vi "D6 Datalog Main.vi"(8 "error in":errorcluster, 11 "Queue Ref":T1) -> ()   [LabVIEW 2022 SP3]
uses:
  Controls/All Queue Ref.ctl
  Controls/D6 Root path.ctl
  Controls/Log main.ctl
  Controls/ALL Health.ctl
  6D_Global.vi
  <vilib>/Waveform/WDTOps.llb/WDT Get Waveform Time Array DBL.vi
  <vilib>/Waveform/DWDTOps.llb/DWDT Get Waveform Time Array.vi
  <vilib>/Waveform/DWDTOps.llb/DWDT Digital to Analog.vi
panel:
  out "error in":errorcluster
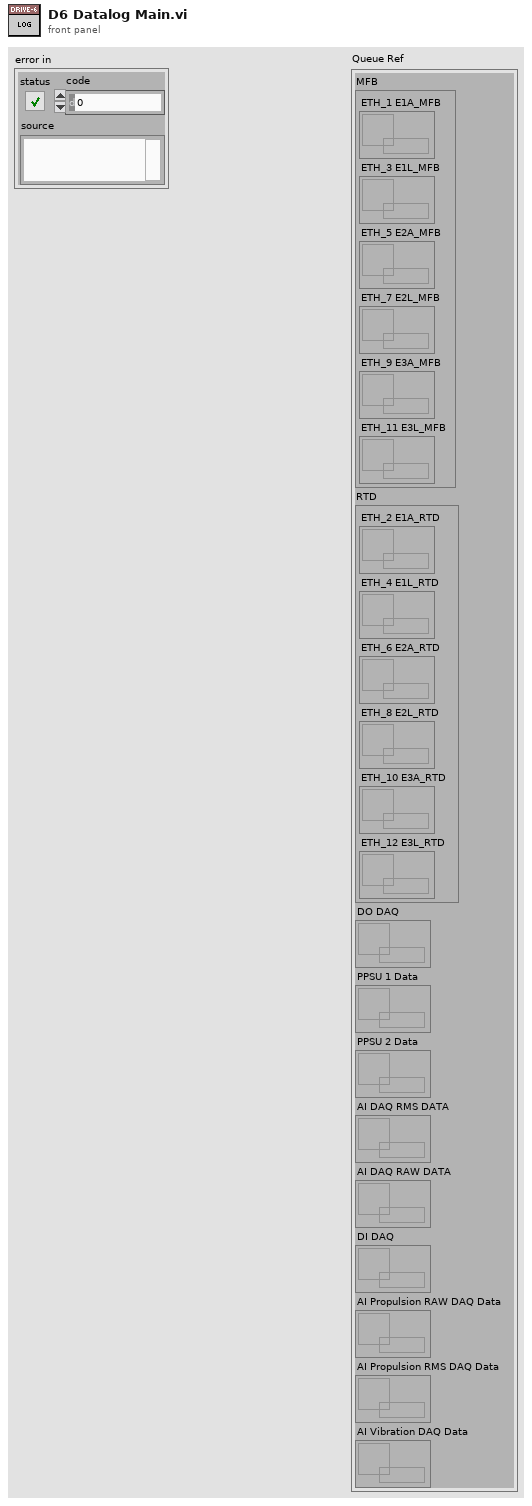
[diagram p1: front panel]
types:
  T1 = typedef "All Queue Ref.ctl" = cluster{"MFB":cluster{"ETH_1 E1A_MFB":refnum<queue>, "ETH_3 E1L_MFB":refnum<queue>, "ETH_5 E2A_MFB":refnum<queue>, "ETH_7 E2L_MFB":refnum<queue>, "ETH_9 E3A_MFB":refnum<queue>, "ETH_11 E3L_MFB":refnum<queue>}, "RTD":cluster{"ETH_2 E1A_RTD ":refnum<queue>, "ETH_4 E1L_RTD ":refnum<queue>, "ETH_6 E2A_RTD ":refnum<queue>, "ETH_8 E2L_RTD ":refnum<queue>, "ETH_10 E3A_RTD ":refnum<queue>, "ETH_12 E3L_RTD ":refnum<queue>}, "DO DAQ":refnum<queue>, "PPSU 1 Data":refnum<queue>, "PPSU 2 Data":refnum<queue>, "AI DAQ RMS DATA":refnum<queue>, "AI DAQ RAW DATA":refnum<queue>, "DI DAQ":refnum<queue>, "AI Propulsion RAW DAQ Data":refnum<queue>, "AI Propulsion RMS DAQ Data":refnum<queue>, "AI Vibration DAQ Data":refnum<queue>}
  T2 = typedef "Log main.ctl" = enum16{"Init", "Poll", "Flush Qs", "Create File", "PPSU Data", "Log MFB", "Log RTD", "Log DO", "Log AI RAW", "Log AI RMS", "Log AI RMS Propulsion", "Log AI RAW Propulsion ", "Log AI Vibration", "Log DI", "Close File", "Error", "Exit"}
  T3 = typedef "D6 Root path.ctl" = cluster{"Data":path, "Sub VI's":path, "Source code":path}
  T4 = cluster{"in progress?":bool, "tdms ref":refnum<k34>, "Start time":timestamp, "Root Path":T3, "Queue Ref":T1}
  T5 = enum16{"open", "open or create", "create or replace", "create", "open (read-only)"}
  T6 = typedef "ALL Health.ctl" = enum16{"AI HS", "AI Vibration HS", "AI Propulsion HS", "DO HS", "Datalog HS", "PPSU HS", "ETH_1 DAQ", "ETH_1 RTD", "ETH_2 DAQ", "ETH_2 RTD", "ETH_5 RTD"}
  T7 = enum16{"Init", "Read 'All'", "Read 'n'", "Read '1'", "Write '1'", "Write 'n'", "Write 'All'"}
  T8 = cluster{"ETH_1 E1A_MFB":refnum<queue>, "ETH_3 E1L_MFB":refnum<queue>, "ETH_5 E2A_MFB":refnum<queue>, "ETH_7 E2L_MFB":refnum<queue>, "ETH_9 E3A_MFB":refnum<queue>, "ETH_11 E3L_MFB":refnum<queue>}
  T9 = cluster{"ETH_2 E1A_RTD ":refnum<queue>, "ETH_4 E1L_RTD ":refnum<queue>, "ETH_6 E2A_RTD ":refnum<queue>, "ETH_8 E2L_RTD ":refnum<queue>, "ETH_10 E3A_RTD ":refnum<queue>, "ETH_12 E3L_RTD ":refnum<queue>}
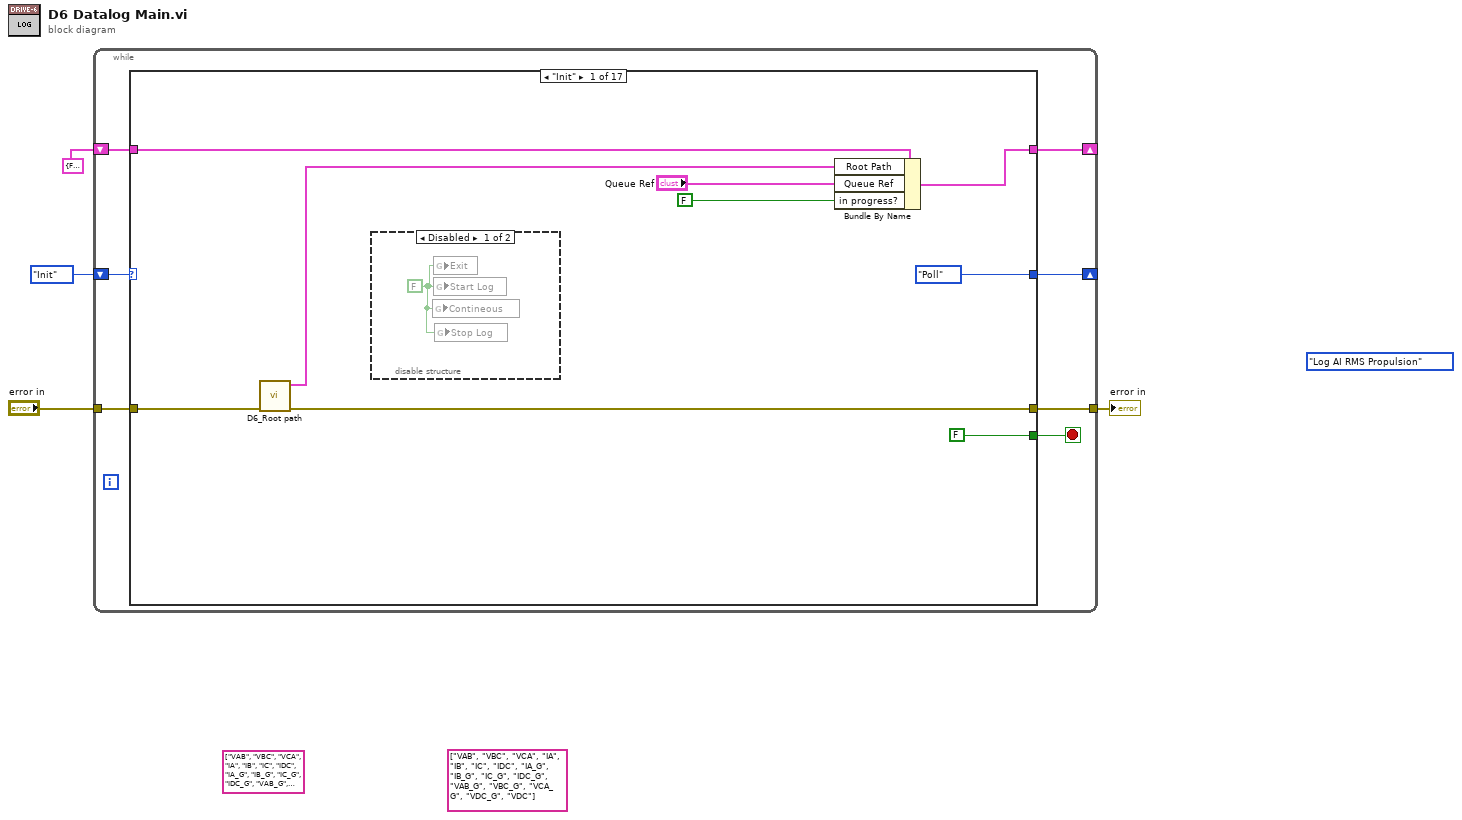
[diagram p0: block diagram]
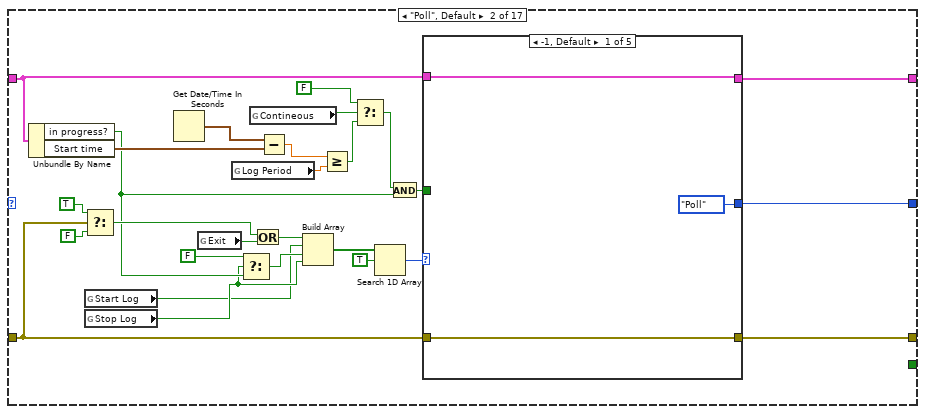
[diagram p3: hidden frame]
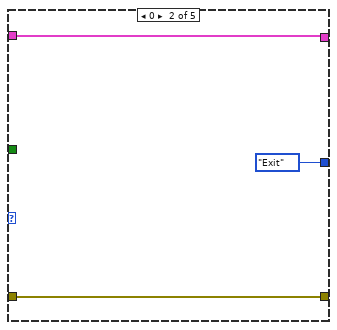
[diagram p4: hidden frame]
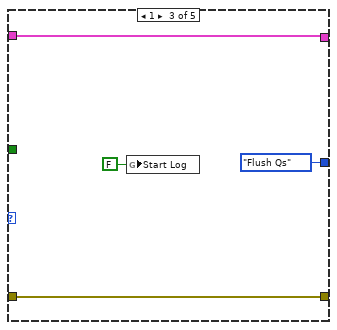
[diagram p5: hidden frame]
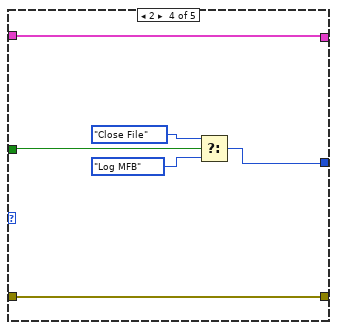
[diagram p6: hidden frame]
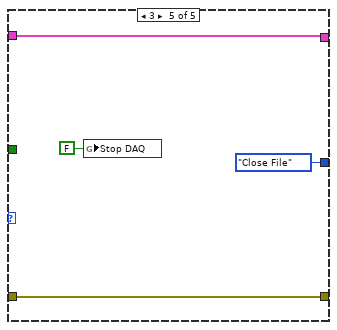
[diagram p7: hidden frame]
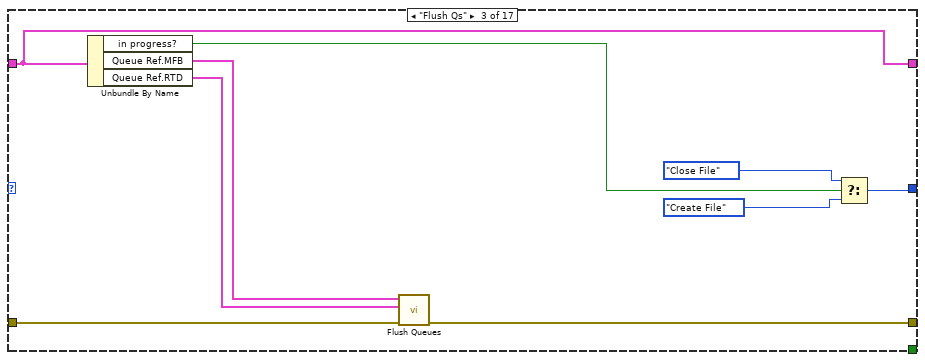
[diagram p8: hidden frame]
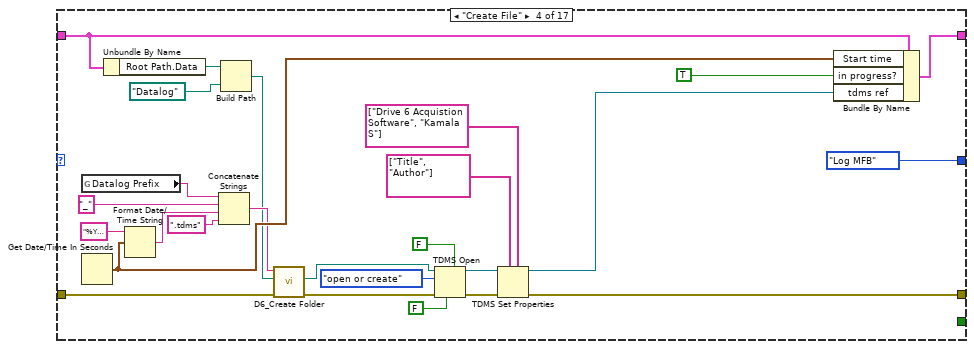
[diagram p9: hidden frame]
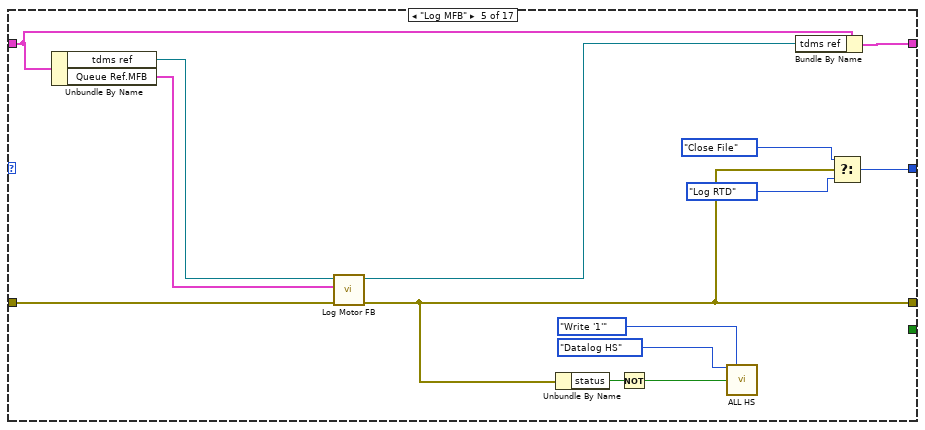
[diagram p10: hidden frame]
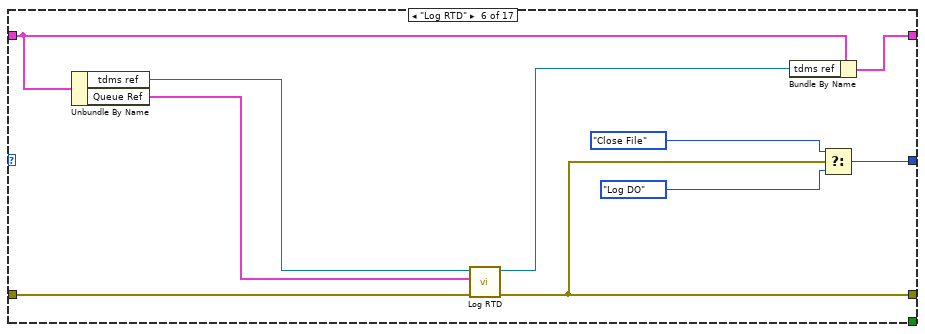
[diagram p11: hidden frame]
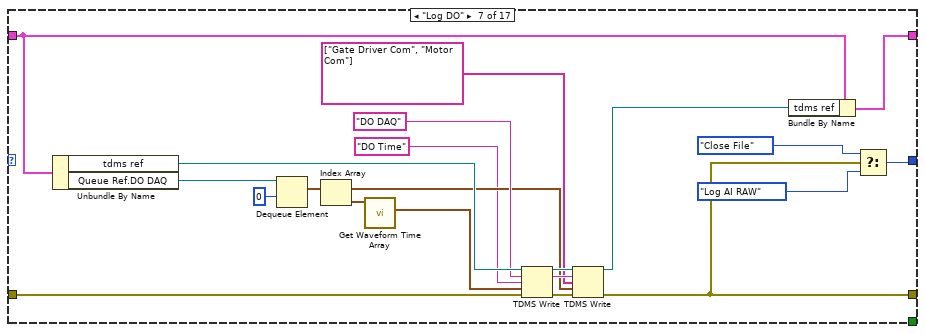
[diagram p12: hidden frame]
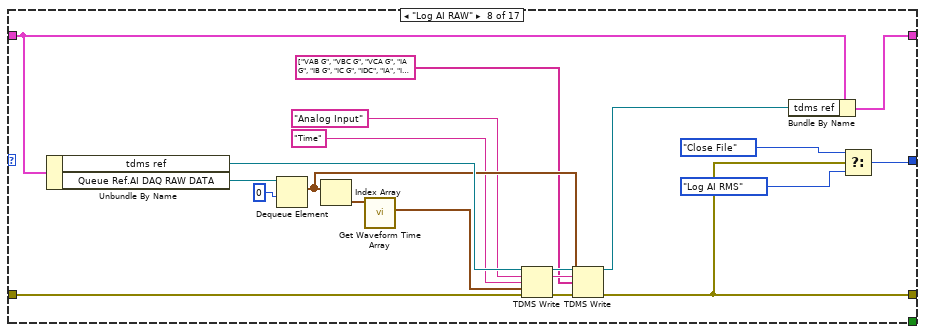
[diagram p13: hidden frame]
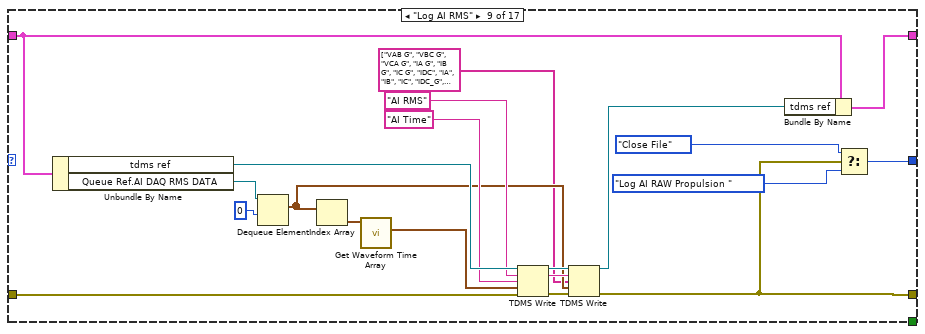
[diagram p14: hidden frame]
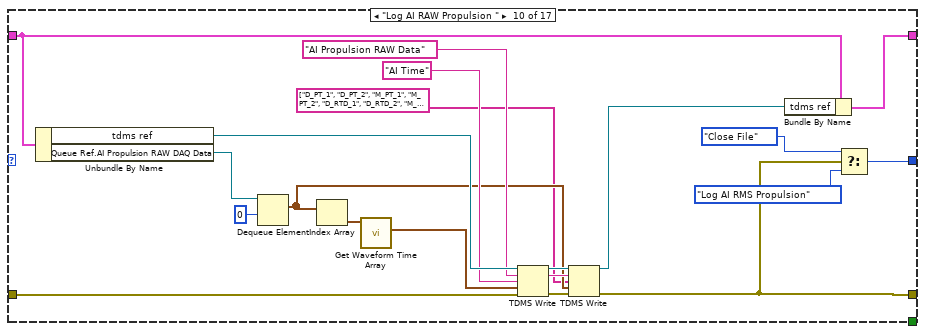
[diagram p15: hidden frame]
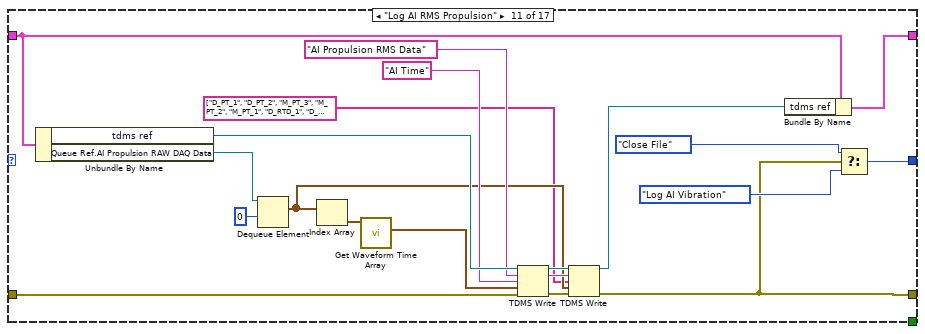
[diagram p16: hidden frame]
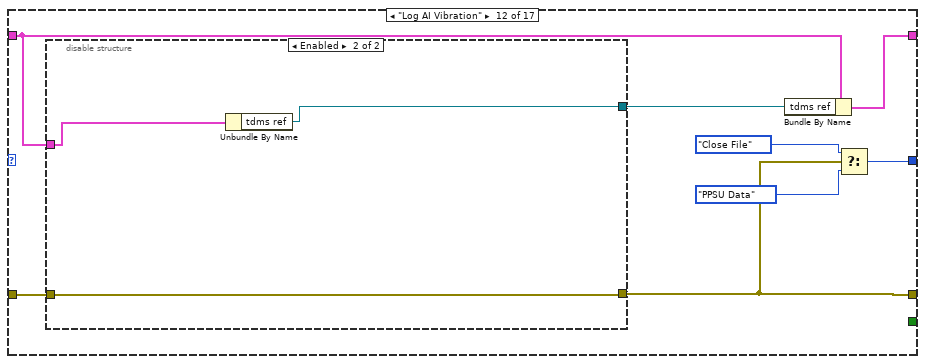
[diagram p17: hidden frame]
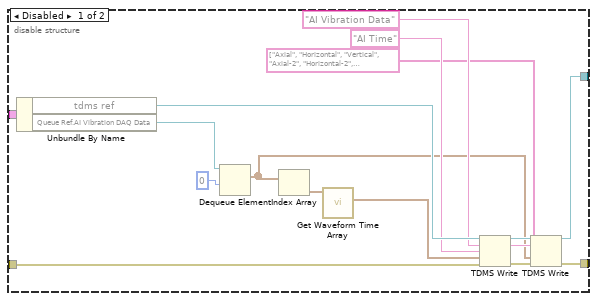
[diagram p18: hidden frame]
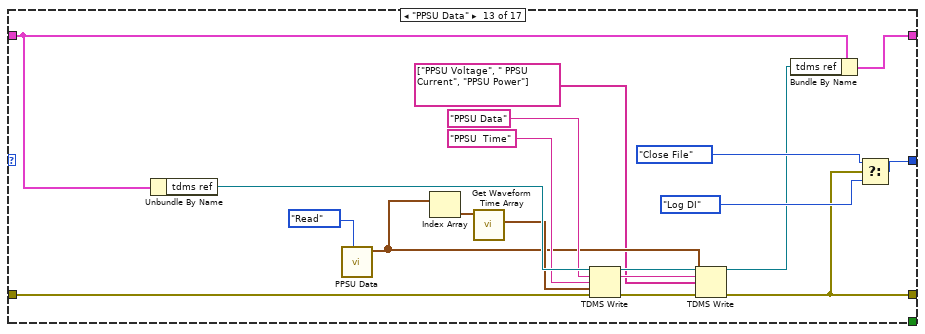
[diagram p19: hidden frame]
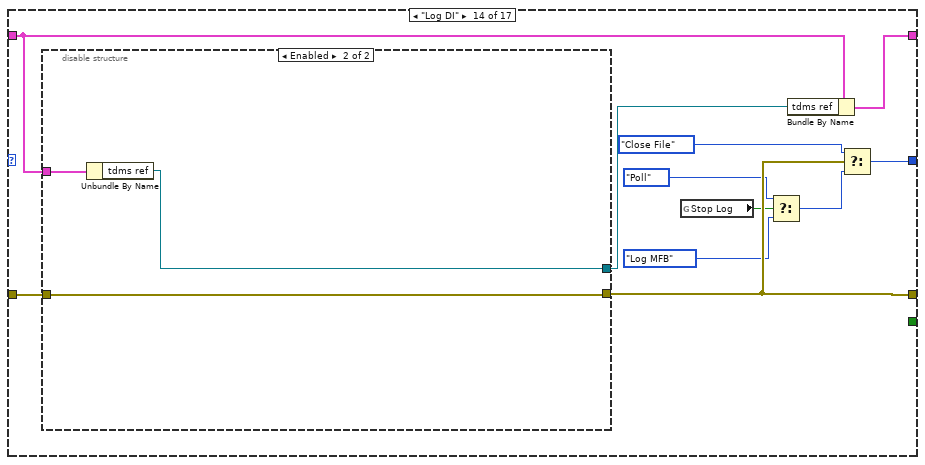
[diagram p20: hidden frame]
diagram:
  (unwired) string[] ["VAB", "VBC", "VCA", "IA", "IB", "IC", "IDC", "IA_G", "IB_G", "IC_G", "IDC_G", "VAB_G", "VBC_G", "VCA_G", "VDC_G", "VDC"] ("channel name(s) in (Untitled)")
  (unwired) string[] ["VAB", "VBC", "VCA", "IA", "IB", "IC", "IDC", "IA_G", "IB_G", "IC_G", "IDC_G", "VAB_G", "VBC_G", "VCA_G", "VDC_G", "VDC"] ("channel name(s) in (Untitled)")
  (unwired) Log_main."Log AI RMS Propulsion"
  n1 = while {
    shift-right: [w10] -> _
    shift-left: Log_main."Init" -> [w11]
    shift-right: [w7] -> _
    shift-left: T4 {"in progress?"=FALSE, "tdms ref"=refnum, "Start time"=timestamp(0 s since 1904-01-01), "Root Path"={"Data"=path "", "Sub VI's"=path "", "Source code"=path ""}, "Queue Ref"={"MFB"={"ETH_1 E1A_MFB"=refnum, "ETH_3 E1L_MFB"=refnum, "ETH_5 E2A_MFB"=refnum, "ETH_7 E2L_MFB"=refnum, "ETH_9 E3A_MFB"=refnum, "ETH_11 E3L_MFB"=refnum}, "RTD"={"ETH_2 E1A_RTD "=refnum, "ETH_4 E1L_RTD "=refnum, "ETH_6 E2A_RTD "=refnum, "ETH_8 E2L_RTD "=refnum, "ETH_10 E3A_RTD "=refnum, "ETH_12 E3L_RTD "=refnum}, "DO DAQ"=refnum, "PPSU 1 Data"=refnum, "PPSU 2 Data"=refnum, "AI DAQ RMS DATA"=refnum, "AI DAQ RAW DATA"=refnum, "DI DAQ"=refnum, "AI Propulsion RAW DAQ Data"=refnum, "AI Propulsion RMS DAQ Data"=refnum, "AI Vibration DAQ Data"=refnum}} -> [w8]
    tunnel: "error in" -> [w6]
    tunnel: [w5] -> w2
    stop <- w9 stop-if-true
    n2 = case shown="\"Init\"" w11 {
      tunnel: [Log_main."Poll" w48 w77 Log_main."Log MFB" w115 w125 w143 w161 w175 w201 w220 w228 w260 w280 Log_main."Exit" w322 Log_main."Close File"] -> w10
      tunnel: [FALSE _ _ _ _ _ _ _ _ _ _ _ _ _ TRUE _ TRUE] -> w9
      tunnel: w8 -> [w19 w45 w75 w90 w116 w126 w146 w164 w177 w203 w222 w230 w259 w279 w311 w324 w335]
      tunnel: [w20 w46 w75 w93 w117 w127 w145 w163 w176 w202 w221 w229 w258 w278 w311 w325 w335] -> w7
      tunnel: w6 -> [w18 w24 w74 w84 w112 w122 w147 w165 w178 w204 w223 w231 w255 w282 w310 w327 w336]
      tunnel: [w16 w47 w71 w78 w106 w121 w141 w159 w179 w205 w224 w232 w261 w281 w310 w326 w336] -> w5
      frame "Init" {
        n3 = call "D6_Root path.vi"("error in (no error)"=w18) -> ("error out"=w16:errorcluster, "Root Path"=w17:T3)  [unwired: 9 in]
        n4 = disable-structure shown="Disabled" {
          frame Disabled {
            w21 = FALSE ("Exit")
            n5 = global write "6D_Global.vi" "Contineous"(w21) -> ()
            n6 = global write "6D_Global.vi" "Exit"(w21) -> ()
            n7 = global write "6D_Global.vi" "Start Log"(w21) -> ()
            n8 = global write "6D_Global.vi" "Stop Log"(w21) -> ()
          }
          frame Enabled {
          }
        }
        n9 = Bundle By Name(cluster=w19, "Root Path"=w17, "Queue Ref"="Queue Ref", "in progress?"=FALSE) -> (w20:T4)
      }
      frame "Poll", Default {
        n10 = Unbundle By Name(w45) -> ("in progress?"=w26:bool, "Start time"=w36:timestamp)
        n11 = Select(t=TRUE, s=w24, f=FALSE) -> (s? t:f=w35:bool)
        n12 = global read "6D_Global.vi" "Start Log"() -> (w22:bool)
        n13 = global read "6D_Global.vi" "Stop Log"() -> (w23:bool)
        n14 = Get Date/Time In Seconds() -> (seconds since 1Jan1904=w37:timestamp)
        n15 = global read "6D_Global.vi" "Exit"() -> (w33:bool)
        n16 = global read "6D_Global.vi" "Log Period"() -> (w32:dbl)
        n17 = Select(t=FALSE ("Stop Log"), s=w23, f=w26) -> (s? t:f=w25:bool)
        n18 = global read "6D_Global.vi" "Contineous"() -> (w31:bool)
        n19 = Or(x=w35, y=w33) -> (x .or. y?=w34:bool)
        n20 = Subtract(x=w37, y=w36) -> (x-y=w39:dbl)
        n21 = Build Array(w34, w22, w25, w23) -> (w42:bool[])
        n22 = Greater Or Equal?(x=w39, y=w32) -> (x >= y?=w30:bool)
        n23 = Select(t=FALSE, s=w31, f=w30) -> (s? t:f=w29:bool)
        n24 = Search 1D Array(1D array=w42, element=TRUE) -> (index of element=w43:i32)  [unwired: 1 in]
        n25 = And(x=w29, y=w26) -> (x .and. y?=w38:bool)
        n26 = case shown="-1, Default" w43 {
          tunnel: [Log_main."Poll" Log_main."Exit" Log_main."Flush Qs" w59 Log_main."Close File"] -> w48
          tunnel: w24 -> [w50 w53 w58 w63 w66]
          tunnel: [w50 w53 w58 w63 w66] -> w47
          tunnel: [w51 w54 w57 w64 w67] -> w46
          tunnel: w45 -> [w51 w54 w57 w64 w67]
          tunnel: w38 -> [_ _ _ w62 _]
          frame -1, Default {
          }
          frame 0 {
          }
          frame 1 {
            n27 = global write "6D_Global.vi" "Start Log"(FALSE ("Start Log")) -> ()
          }
          frame 2 {
            n28 = Select(t=Log_main."Close File", s=w62, f=Log_main."Log MFB") -> (s? t:f=w59:T2)
          }
          frame 3 {
            n29 = global write "6D_Global.vi" "Stop DAQ"(FALSE ("Stop DAQ")) -> ()
          }
        }
      }
      frame "Flush Qs" {
        n30 = Unbundle By Name(w75) -> ("in progress?"=w76:bool, "Queue Ref.MFB"=w73:T8, "Queue Ref.RTD"=w72:T9)
        n31 = call "Flush Queues.vi"("error in"=w74, "RTD"=w72, "MFB"=w73) -> ("error out"=w71:errorcluster)  [unwired: 8 in]
        n32 = Select(t=Log_main."Close File", s=w76, f=Log_main."Create File") -> (s? t:f=w77:T2)
      }
      frame "Create File" {
        n33 = global read "6D_Global.vi" "Datalog Prefix"() -> (w85:string)
        n34 = Get Date/Time In Seconds() -> (seconds since 1Jan1904=w87:timestamp)
        n35 = Unbundle By Name(w90) -> ("Root Path.Data"=w89:path)
        n36 = Format Date/Time String(time format string (%c)="%Y_%b_%d_%Hh_%Mm_%Ssec", seconds (now)=w87) -> (date/time string=w97:string)  [unwired: 1 in]
        n37 = Concatenate Strings(w85, "_" ("string"), w97, ".tdms" ("string")) -> (w82:string)
        n38 = Build Path(base path=w89, name or relative path=path "Datalog" ("base path")) -> (appended path=w81:path)
        n39 = call "D6_Create Folder.vi"("error in (no error)"=w84, "Base Path"=w81, "File Name"=w82) -> ("error out"=w83:errorcluster, "Result File path"=w80:path)  [unwired: 6 in, 1 out]
        n40 = TDMS Open(5:FALSE ("create index file? (T)"), 6:FALSE ("disable buffering? (T)"), 8:w83, 10:T5."open or create" ("operation (0:open)"), 11:w80) -> (0:w102:errorcluster, 3:w103:refnum<k34>)  [unwired: 2 in]
        n41 = TDMS Set Properties(5:string[] ["Drive 6 Acquistion Software", "Kamala S"] ("property names"), 7:string[] ["Title", "Author"] ("property names"), 8:w102, 11:w103) -> (0:w78:errorcluster, 3:w91:refnum<k34>)  [unwired: 4 out]
        n42 = Bundle By Name(cluster=w90, "Start time"=w87, "in progress?"=TRUE, "tdms ref"=w91) -> (w93:T4)
      }
      frame "Log MFB" {
        n43 = Unbundle By Name(w116) -> ("tdms ref"=w111:refnum<k34>, "Queue Ref.MFB"=w109:T8)
        n44 = call "Log Motor FB.vi"("error in"=w112, "MFB"=w109, "tdms file in"=w111) -> ("error out"=w106:errorcluster, "tdms file in"=w110:refnum<k34>)  [unwired: 7 in]
        n45 = Unbundle By Name(w106) -> ("status"=w105:bool)
        n46 = Not(x=w105) -> (.not. x?=w104:bool)
        n47 = call "ALL HS.vi"("Loop"=ALL_Health."Datalog HS", "Option"=T7."Write '1'", "Status"=w104) -> ()  [unwired: 10 in, 3 out]
        n48 = Bundle By Name(cluster=w116, "tdms ref"=w110) -> (w117:T4)
        n49 = Select(t=Log_main."Close File", s=w106, f=Log_main."Log RTD") -> (s? t:f=w115:T2)
      }
      frame "Log RTD" {
        n50 = Unbundle By Name(w126) -> ("tdms ref"=w120:refnum<k34>, "Queue Ref"=w118:T1)
        n51 = call "Log RTD.vi"("error in 2"=w122, "Queue Ref"=w118, "tdms file in 2"=w120) -> ("error out 2"=w121:errorcluster, "tdms file in"=w119:refnum<k34>)  [unwired: 7 in]
        n52 = Bundle By Name(cluster=w126, "tdms ref"=w119) -> (w127:T4)
        n53 = Select(t=Log_main."Close File", s=w121, f=Log_main."Log DO") -> (s? t:f=w125:T2)
      }
      frame "Log DO" {
        n54 = Unbundle By Name(w146) -> ("tdms ref"=w139:refnum<k34>, "Queue Ref.DO DAQ"=w138:refnum<queue>)
        n55 = Dequeue Element(queue=w138, timeout in ms (-1)=0) -> (element=w130:waveform(dbl)[])  [unwired: 1 in, 3 out]
        n56 = Index Array(array=w130) -> (element=w137:waveform(dbl))  [unwired: 1 in]
        n57 = call-poly <vilib>:"Get Waveform Time Array.vi"("waveform in"=w137) -> ("X array"=w135:timestamp[])  [unwired: 9 in, 1 out]
        n58 = TDMS Write(0:w139, 5:"DO DAQ" ("group name in (Untitled)"), 7:"DO Time" ("group name in (Untitled)"), 9:w135, 11:w147) -> (4:w133:refnum<k34>, 6:w136:string, 15:w134:errorcluster)  [unwired: 1 in, 1 out]
        n59 = TDMS Write(0:w133, 5:w136, 7:string[] ["Gate Driver Com", "Motor Com"] ("channel name(s) in (Untitled)"), 9:w130, 11:w134) -> (4:w144:refnum<k34>, 15:w141:errorcluster)  [unwired: 1 in, 2 out]
        n60 = Bundle By Name(cluster=w146, "tdms ref"=w144) -> (w145:T4)
        n61 = Select(t=Log_main."Close File", s=w141, f=Log_main."Log AI RAW") -> (s? t:f=w143:T2)
      }
      frame "Log AI RAW" {
        n62 = Unbundle By Name(w164) -> ("tdms ref"=w167:refnum<k34>, "Queue Ref.AI DAQ RAW DATA"=w166:refnum<queue>)
        n63 = Dequeue Element(queue=w166, timeout in ms (-1)=0) -> (element=w152:waveform(dbl)[])  [unwired: 1 in, 3 out]
        n64 = Index Array(array=w152) -> (element=w158:waveform(dbl))  [unwired: 1 in]
        n65 = call-poly <vilib>:"Get Waveform Time Array.vi"("waveform in"=w158) -> ("X array"=w156:timestamp[])  [unwired: 9 in, 1 out]
        n66 = TDMS Write(0:w167, 5:"Analog Input" ("group name in (Untitled)"), 7:"Time" ("group name in (Untitled)"), 9:w156, 11:w165) -> (4:w154:refnum<k34>, 6:w157:string, 15:w155:errorcluster)  [unwired: 1 in, 1 out]
        n67 = TDMS Write(0:w154, 5:w157, 7:string[] ["VAB G", "VBC G", "VCA G", "IA G", "IB G", "IC G", "IDC", "IA", "IB", "IC", "IDC_G", "VAB", "VBC", "VCA", "VDC_G", "VDC"] ("channel name(s) in (Untitled)"), 9:w152, 11:w155) -> (4:w162:refnum<k34>, 15:w159:errorcluster)  [unwired: 1 in, 2 out]
        n68 = Bundle By Name(cluster=w164, "tdms ref"=w162) -> (w163:T4)
        n69 = Select(t=Log_main."Close File", s=w159, f=Log_main."Log AI RMS") -> (s? t:f=w161:T2)
      }
      frame "Log AI RMS" {
        n70 = Unbundle By Name(w177) -> ("tdms ref"=w187:refnum<k34>, "Queue Ref.AI DAQ RMS DATA"=w171:refnum<queue>)
        n71 = Dequeue Element(queue=w171, timeout in ms (-1)=0) -> (element=w170:waveform(dbl)[])  [unwired: 1 in, 3 out]
        n72 = Index Array(array=w170) -> (element=w184:waveform(dbl))  [unwired: 1 in]
        n73 = call-poly <vilib>:"Get Waveform Time Array.vi"("waveform in"=w184) -> ("X array"=w182:timestamp[])  [unwired: 9 in, 1 out]
        n74 = TDMS Write(0:w187, 5:"AI RMS" ("group name in (Untitled)"), 7:"AI Time" ("group name in (Untitled)"), 9:w182, 11:w178) -> (4:w180:refnum<k34>, 6:w183:string, 15:w181:errorcluster)  [unwired: 1 in, 1 out]
        n75 = TDMS Write(0:w180, 5:w183, 7:string[] ["VAB G", "VBC G", "VCA G", "IA G", "IB G", "IC G", "IDC", "IA", "IB", "IC", "IDC_G", "VAB", "VBC", "VCA", "VDC_G", "VDC"] ("channel name(s) in (Untitled)"), 9:w170, 11:w181) -> (4:w186:refnum<k34>, 15:w179:errorcluster)  [unwired: 1 in, 2 out]
        n76 = Bundle By Name(cluster=w177, "tdms ref"=w186) -> (w176:T4)
        n77 = Select(t=Log_main."Close File", s=w179, f=Log_main."Log AI RAW Propulsion ") -> (s? t:f=w175:T2)
      }
      frame "Log AI RAW Propulsion " {
        n78 = Unbundle By Name(w203) -> ("tdms ref"=w199:refnum<k34>, "Queue Ref.AI Propulsion RAW DAQ Data"=w190:refnum<queue>)
        n79 = Dequeue Element(queue=w190, timeout in ms (-1)=0) -> (element=w189:waveform(dbl)[])  [unwired: 1 in, 3 out]
        n80 = Index Array(array=w189) -> (element=w198:waveform(dbl))  [unwired: 1 in]
        n81 = call-poly <vilib>:"Get Waveform Time Array.vi"("waveform in"=w198) -> ("X array"=w196:timestamp[])  [unwired: 9 in, 1 out]
        n82 = TDMS Write(0:w199, 5:"AI Propulsion RAW Data" ("group name in (Untitled)"), 7:"AI Time" ("group name in (Untitled)"), 9:w196, 11:w204) -> (4:w194:refnum<k34>, 6:w197:string, 15:w195:errorcluster)  [unwired: 1 in, 1 out]
        n83 = TDMS Write(0:w194, 5:w197, 7:string[] ["D_PT_1", "D_PT_2", "M_PT_1", "M_PT_2", "D_RTD_1", "D_RTD_2", "M_RTD_1", "M_RTD_2", "M_RTD_3", "M_PT_3"] ("channel name(s) in (Untitled)"), 9:w189, 11:w195) -> (4:w207:refnum<k34>, 15:w205:errorcluster)  [unwired: 1 in, 2 out]
        n84 = Bundle By Name(cluster=w203, "tdms ref"=w207) -> (w202:T4)
        n85 = Select(t=Log_main."Close File", s=w205, f=Log_main."Log AI RMS Propulsion") -> (s? t:f=w201:T2)
      }
      frame "Log AI RMS Propulsion" {
        n86 = Unbundle By Name(w222) -> ("tdms ref"=w219:refnum<k34>, "Queue Ref.AI Propulsion RAW DAQ Data"=w210:refnum<queue>)
        n87 = Dequeue Element(queue=w210, timeout in ms (-1)=0) -> (element=w209:waveform(dbl)[])  [unwired: 1 in, 3 out]
        n88 = Index Array(array=w209) -> (element=w218:waveform(dbl))  [unwired: 1 in]
        n89 = call-poly <vilib>:"Get Waveform Time Array.vi"("waveform in"=w218) -> ("X array"=w216:timestamp[])  [unwired: 9 in, 1 out]
        n90 = TDMS Write(0:w219, 5:"AI Propulsion RMS Data" ("group name in (Untitled)"), 7:"AI Time" ("group name in (Untitled)"), 9:w216, 11:w223) -> (4:w214:refnum<k34>, 6:w217:string, 15:w215:errorcluster)  [unwired: 1 in, 1 out]
        n91 = TDMS Write(0:w214, 5:w217, 7:string[] ["D_PT_1", "D_PT_2", "M_PT_3", "M_PT_2", "M_PT_1", "D_RTD_1", "D_RTD_2", "M_RTD_3", "M_RTD_2", "M_RTD_1"] ("channel name(s) in (Untitled)"), 9:w209, 11:w215) -> (4:w227:refnum<k34>, 15:w224:errorcluster)  [unwired: 1 in, 2 out]
        n92 = Bundle By Name(cluster=w222, "tdms ref"=w227) -> (w221:T4)
        n93 = Select(t=Log_main."Close File", s=w224, f=Log_main."Log AI Vibration") -> (s? t:f=w220:T2)
      }
      frame "Log AI Vibration" {
        n94 = disable-structure shown="Enabled" {
          disable-tunnel: [w251 w253] -> w235
          disable-tunnel: [w250 w252] -> w232
          disable-tunnel: w231 -> [w249 w252]
          disable-tunnel: w230 -> [w248 w254]
          frame Disabled {
            n95 = Unbundle By Name(w248) -> ("tdms ref"=w247:refnum<k34>, "Queue Ref.AI Vibration DAQ Data"=w238:refnum<queue>)
            n96 = Dequeue Element(queue=w238, timeout in ms (-1)=0) -> (element=w237:waveform(dbl)[])  [unwired: 1 in, 3 out]
            n97 = Index Array(array=w237) -> (element=w246:waveform(dbl))  [unwired: 1 in]
            n98 = call-poly <vilib>:"Get Waveform Time Array.vi"("waveform in"=w246) -> ("X array"=w244:timestamp[])  [unwired: 9 in, 1 out]
            n99 = TDMS Write(0:w247, 5:"AI Vibration Data" ("group name in (Untitled)"), 7:"AI Time" ("group name in (Untitled)"), 9:w244, 11:w249) -> (4:w242:refnum<k34>, 6:w245:string, 15:w243:errorcluster)  [unwired: 1 in, 1 out]
            n100 = TDMS Write(0:w242, 5:w245, 7:string[] ["Axial", "Horizontal", "Vertical", "Axial-2", "Horizontal-2", "Vertical-2"] ("channel name(s) in (Untitled)"), 9:w237, 11:w243) -> (4:w251:refnum<k34>, 15:w250:errorcluster)  [unwired: 1 in, 2 out]
          }
          frame Enabled {
            n101 = Unbundle By Name(w254) -> ("tdms ref"=w253:refnum<k34>)
          }
        }
        n102 = Bundle By Name(cluster=w230, "tdms ref"=w235) -> (w229:T4)
        n103 = Select(t=Log_main."Close File", s=w232, f=Log_main."PPSU Data") -> (s? t:f=w228:T2)
      }
      frame "PPSU Data" {
        n104 = Unbundle By Name(w259) -> ("tdms ref"=w273:refnum<k34>)
        n105 = call "PPSU Data.vi"("Write/Read"=enum16{"Write", "Read"}."Read") -> ("Array"=w264:waveform(dbl)[])  [unwired: 10 in]
        n106 = Index Array(array=w264) -> (element=w272:waveform(dbl))  [unwired: 1 in]
        n107 = call-poly <vilib>:"Get Waveform Time Array.vi"("waveform in"=w272) -> ("X array"=w270:timestamp[])  [unwired: 9 in, 1 out]
        n108 = TDMS Write(0:w273, 5:"PPSU Data" ("group name in (Untitled)"), 7:"PPSU  Time" ("group name in (Untitled)"), 9:w270, 11:w255) -> (4:w268:refnum<k34>, 6:w271:string, 15:w269:errorcluster)  [unwired: 1 in, 1 out]
        n109 = TDMS Write(0:w268, 5:w271, 7:string[] ["PPSU Voltage", " PPSU Current", "PPSU Power"] ("appended array"), 9:w264, 11:w269) -> (4:w257:refnum<k34>, 15:w261:errorcluster)  [unwired: 1 in, 2 out]
        n110 = Bundle By Name(cluster=w259, "tdms ref"=w257) -> (w258:T4)
        n111 = Select(t=Log_main."Close File", s=w261, f=Log_main."Log DI") -> (s? t:f=w260:T2)
      }
      frame "Log DI" {
        n112 = disable-structure shown="Enabled" {
          disable-tunnel: [w299 w306] -> w284
          disable-tunnel: w282 -> [w293 w305]
          disable-tunnel: [w292 w305] -> w281
          disable-tunnel: w279 -> [w288 w307]
          frame Disabled {
            n113 = Unbundle By Name(w288) -> ("tdms ref"=w301:refnum<k34>, "Queue Ref.DI DAQ"=w300:refnum<queue>)
            n114 = Dequeue Element(queue=w300, timeout in ms (-1)=0) -> (element=w290:digitalwaveform[])  [unwired: 1 in, 3 out]
            n115 = Index Array(array=w290) -> (element=w298:digitalwaveform)  [unwired: 1 in]
            n116 = for {
              tunnel: w290 -> [w304] mode=indexing
              tunnel: [w303] -> w289 mode=indexing
              w302 = u16 0 items=["unsigned binary", "offset binary", "2's complement"] ("data format (offset binary)")
              n117 = call-poly <vilib>:"Digital to Analog.vi"("data format (offset binary)"=w302, "digital waveform"=w304) -> ("analog waveform"=w303:waveform(dbl))  [unwired: 6 in, 3 out]
            }
            n118 = call-poly <vilib>:"Get Waveform Time Array.vi"("waveform in"=w298) -> ("X array"=w291:timestamp[])  [unwired: 9 in, 1 out]
            n119 = TDMS Write(0:w301, 5:"Digital Input" ("group name in (Untitled)"), 7:"DI Timestamp" ("group name in (Untitled)"), 9:w291, 11:w293) -> (4:w295:refnum<k34>, 6:w297:string, 15:w296:errorcluster)  [unwired: 1 in, 1 out]
            n120 = TDMS Write(0:w295, 5:w297, 7:string[] ["Ha", "Hb", "Hc", "Ha_G", "Hb_G", "Hc_G"] ("channel name(s) in (Untitled)"), 9:w289, 11:w296) -> (4:w299:refnum<k34>, 15:w292:errorcluster)  [unwired: 1 in, 2 out]
          }
          frame Enabled {
            n121 = Unbundle By Name(w307) -> ("tdms ref"=w306:refnum<k34>)
          }
        }
        n122 = global read "6D_Global.vi" "Stop Log"() -> (w277:bool)
        n123 = Select(t=Log_main."Poll", s=w277, f=Log_main."Log MFB") -> (s? t:f=w274:T2)
        n124 = Bundle By Name(cluster=w279, "tdms ref"=w284) -> (w278:T4)
        n125 = Select(t=Log_main."Close File", s=w281, f=w274) -> (s? t:f=w280:T2)
      }
      frame "Exit" {
      }
      frame "Close File" {
        n126 = Unbundle By Name(w324) -> ("tdms ref"=w329:refnum<k34>)
        n127 = Not A Number/Path/Refnum?(number/path/refnum=w329) -> (NaN/Path/Refnum?=w328:bool)
        n128 = case shown="False" w328 {
          tunnel: [w332 w333] -> w326
          tunnel: w329 -> [w331 _]
          tunnel: w327 -> [w330 w333]
          frame False {
            # "Closing the TDMS file"
            n129 = TDMS Close(8:w330, 11:w331) -> (0:w332:errorcluster)  [unwired: 1 out]
          }
          frame True {
          }
        }
        n130 = call "ALL HS.vi"("Loop"=ALL_Health."Datalog HS", "Option"=T7."Write '1'", "Status"=FALSE) -> ()  [unwired: 10 in, 3 out]
        n131 = global read "6D_Global.vi" "Contineous"() -> (w320:bool)
        n132 = global read "6D_Global.vi" "Exit"() -> (w318:bool)
        n133 = Bundle By Name(cluster=w324, "tdms ref"=refnum<k34> refnum, "in progress?"=FALSE ("f")) -> (w325:T4)
        n134 = Select(t=Log_main."Exit", s=w318, f=Log_main."Poll") -> (s? t:f=w315:T2)
        n135 = Select(t=Log_main."Poll", s=w320, f=w315) -> (s? t:f=w322:T2)
      }
      frame "Error" {
      }
    }
  }
  "error in" <- w2
